vi "demux1_10(x6)_separated.vi"(7 "Mem_mapping in":u16[](array[numeric]), 8 "Boolean array 14":bool[](array[boolean]), 9 "Boolean array 13":bool[](array[boolean]), 10 "Boolean array 12":bool[](array[boolean]), 11 "Boolean array 11":bool[](array[boolean])) -> (0 "output array 14":bool[](array[boolean]), 1 "output array 13":bool[](array[boolean]), 2 "output array 12":bool[](array[boolean]), 3 "output array 11":bool[](array[boolean]))   [LabVIEW 2018, in "MB Relay.lvlib"]
uses:
  MB Relay.lvlib
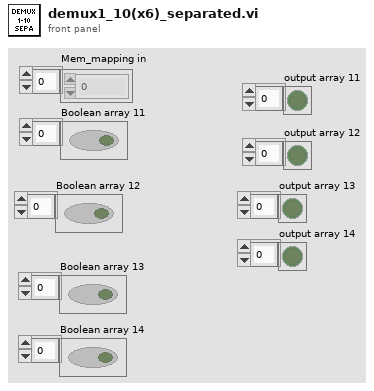
[diagram p1: front panel]
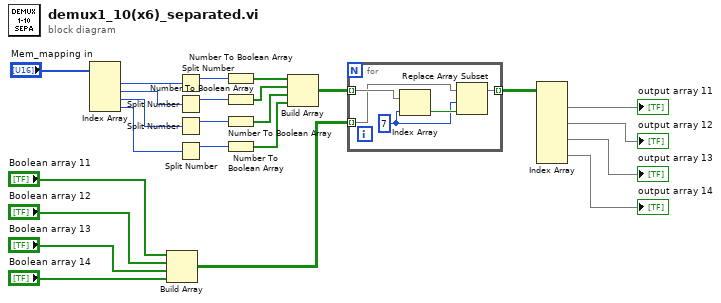
[diagram p0: block diagram]
diagram:
  n1 = Index Array(array="Mem_mapping in") -> (element #1=w24:u16, element #2=w21:u16, element #3=w19:u16, element #4=w17:u16)  [unwired: 4 in]
  n2 = Build Array("Boolean array 11", "Boolean array 12", "Boolean array 13", "Boolean array 14") -> (w6:bool[][])
  n3 = Split Number(x=w24) -> (hi(x)=w23:u8)  [unwired: 1 out]
  n4 = Split Number(x=w21) -> (hi(x)=w22:u8)  [unwired: 1 out]
  n5 = Split Number(x=w19) -> (hi(x)=w20:u8)  [unwired: 1 out]
  n6 = Split Number(x=w17) -> (hi(x)=w18:u8)  [unwired: 1 out]
  n7 = Number To Boolean Array(number=w23) -> (Boolean array=w11:bool[])
  n8 = Number To Boolean Array(number=w22) -> (Boolean array=w10:bool[])
  n9 = Number To Boolean Array(number=w20) -> (Boolean array=w9:bool[])
  n10 = Number To Boolean Array(number=w18) -> (Boolean array=w8:bool[])
  n11 = Build Array(w11, w10, w9, w8) -> (w7:bool[][])
  n12 = for {
    tunnel: w7 -> [w28] mode=indexing
    tunnel: w6 -> [w26] mode=indexing
    tunnel: [w25] -> w5 mode=indexing
    w27 = 7 ("index")
    n13 = Index Array(array=w28, index=w27) -> (element=w29:bool)
    n14 = Replace Array Subset(array=w26, new element=w29, index=w27) -> (w25:bool[])
  }
  n15 = Index Array(array=w5) -> (element #1=→"output array 11":bool[], element #2=→"output array 12":bool[], element #3=→"output array 13":bool[], element #4=→"output array 14":bool[])  [unwired: 8 in]
